vi "StopImageAcquisition.vi"(11 "camera queue":refnum<queue>) -> ()   [LabVIEW 2011]
uses:
  CmdData_NewFrame.ctl
  <vilib>/vision/Image Controls.llb/IMAQ Image.ctl
  CmdEnum_CameraFrameType.ctl
  CmdEnum_CameraIn.ctl
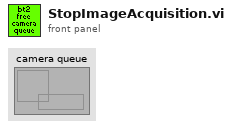
[diagram p1: front panel]
types:
  T1 = typedef "CmdEnum_CameraIn.ctl" = enum32{"Init", "Close", "ShowSettingsDialog", "EndGrab", "GrabZLUT", "GrabToTracker", "GrabToQueue", "AdjustROIs"}
  T2 = typedef "CmdData_NewFrame.ctl" = cluster{"Buffer Image":T3, "Frame #":i32, "Hardware ROI Index":i32, "Timestamp":dbl, "Type":T4}
  T3 = typedef "IMAQ Image.ctl" = refnum<image>
  T4 = typedef "CmdEnum_CameraFrameType.ctl" = enum16{"Full", "HardwareROI", "EndGrabMarker"}
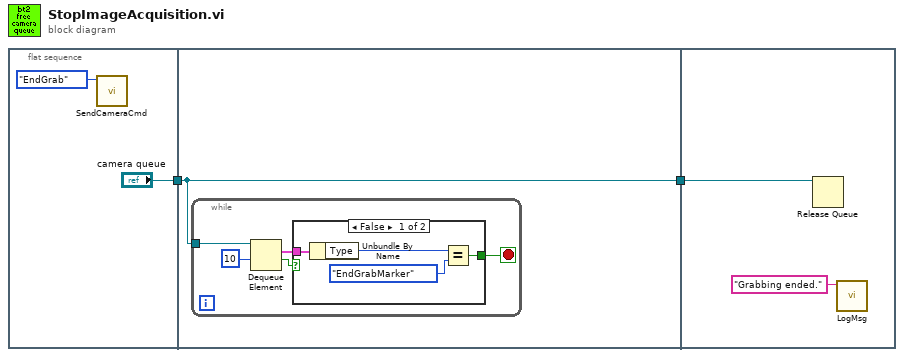
[diagram p0: block diagram]
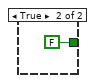
[diagram p2: hidden frame]
diagram:
  n1 = flat-sequence {
    tunnel: ["camera queue"] -> w2
    tunnel: w2 -> [w5]
    tunnel: [w5] -> w1
    tunnel: w1 -> [w17]
    frame #0 {
      n2 = call "SendCameraCmd.vi"("Camera cmd (SettingsDlg)"=CmdEnum_CameraIn."EndGrab") -> ()  [unwired: 11 in]
    }
    frame #1 {
      n3 = while {
        tunnel: w5 -> [w9]
        stop <- w6 stop-if-true
        n4 = Dequeue Element(queue=w9, timeout in ms (-1)=10) -> (element=w7:T2, timed out?=w8:bool)  [unwired: 1 in, 2 out]
        n5 = case shown="False" w8 {
          tunnel: w7 -> [w14 _]
          tunnel: [w11 FALSE] -> w6
          frame False {
            n6 = Unbundle By Name(w14) -> ("Type"=w13:T4)
            n7 = Equal?(x=w13, y=enum16{"Full", "HardwareROI", "EndGrabMarker"}."EndGrabMarker") -> (x = y?=w11:bool)
          }
          frame True {
          }
        }
      }
    }
    frame #2 {
      n8 = Release Queue(queue=w17) -> ()  [unwired: 2 in, 3 out]
      n9 = call "LogMsg.vi"("msg"="Grabbing ended.") -> ()  [unwired: 11 in]
    }
  }
